vi "Ground1287.vi"(2 "Error In (No Error)":errorcluster, 3 "VISA Name In":refnum<visa-resource-name>="Solartron1287") -> (0 "Error Out":errorcluster, 1 "VISA Name Out":refnum<visa-resource-name>)   [LabVIEW 2018]
panel:
  # "Inputs"
  # "Outputs"
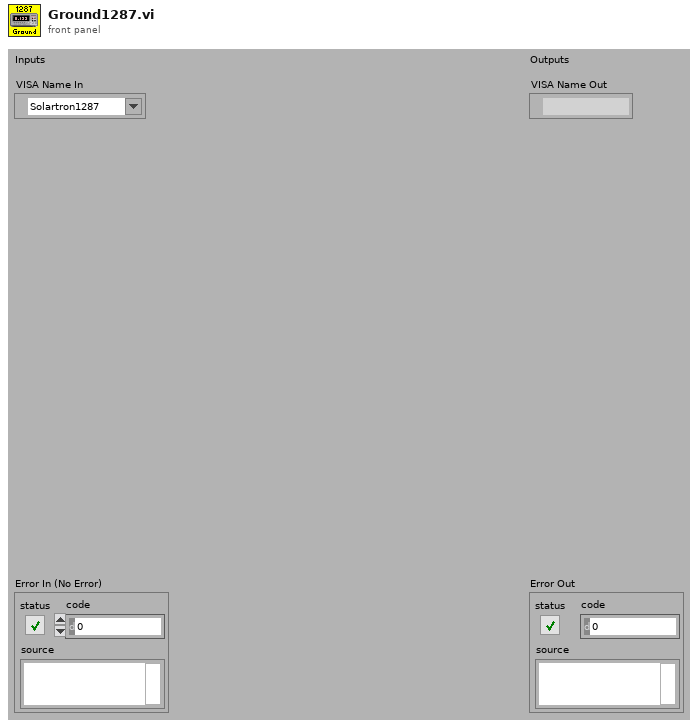
[diagram p1: front panel]
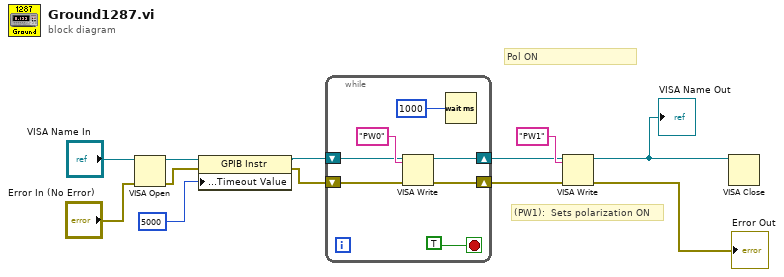
[diagram p0: block diagram]
diagram:
  # "Pol ON"
  # "(PW1):  Sets polarization ON"
  n1 = VISA Open(error in (no error)="Error In (No Error)", VISA resource name="VISA Name In") -> (VISA resource name=w10:refnum<visa-resource-name>, error out=w9:errorcluster)  [unwired: 3 in]
  n2 = property class="GPIB Instr"(reference=w10, error in=w9, "General Settings:Timeout Value"=u32 5000) -> (reference out=w4:refnum<visa-resource-name>, error out=w3:errorcluster)
  n3 = while {
    shift-right: [w16] -> w2
    shift-left: w4 -> [w18]
    shift-right: [w15] -> w1
    shift-left: w3 -> [w17]
    stop <- TRUE stop-if-true
    n4 = VISA Write(VISA resource name=w18, write buffer="PW0", error in (no error)=w17) -> (VISA resource name out=w16:refnum<visa-resource-name>, error out=w15:errorcluster)  [unwired: 1 out]
    n5 = Wait (ms)(milliseconds to wait=1000) -> ()  [unwired: 1 out]
  }
  n6 = VISA Write(VISA resource name=w2, write buffer="PW1", error in (no error)=w1) -> (VISA resource name out=w7:refnum<visa-resource-name>, error out=→"Error Out":errorcluster)  [unwired: 1 out]
  "VISA Name Out" <- w7
  n7 = VISA Close(VISA resource name=w7) -> ()  [unwired: 1 in, 1 out]
